vi "testIgnores Label Marker In Middle of Argument.vi"(8 "error in (no error)":errorcluster, 11 "TestCase in":refnum<class "Options Parsing Tests.lvclass">) -> (0 "error out":errorcluster, 3 "TestCase out":refnum<class "Options Parsing Tests.lvclass">)   [LabVIEW 2011, in "Options Parsing Tests.lvclass"]
uses:
  Options Parsing Tests.lvclass
  Argument Parser/Option Class/Option Configuration.ctl
  Argument Parser/Option Class/Argument Type.ctl
  <vilib>/addons/_JKI Toolkits/VI Tester/TestCase.llb/TestCase.lvclass
  Argument Parser/Option Set Class/Option Set.lvclass
  Argument Parser/Option Class/Option.lvclass
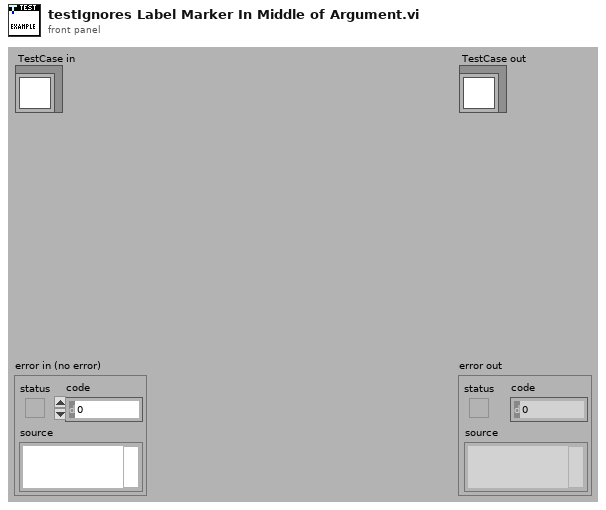
[diagram p1: front panel]
types:
  T1 = typedef "Option Parser.lvlib/Option.lvclass/Option Configuration.ctl" = cluster{"Option Type":T2, "Option Labels":string[], "Key":string, "Description":string, "Required":bool, "Default Value":string}
  T2 = typedef "Option Parser.lvlib/Option.lvclass/Argument Type.ctl" = enum16{"flag", "value"}
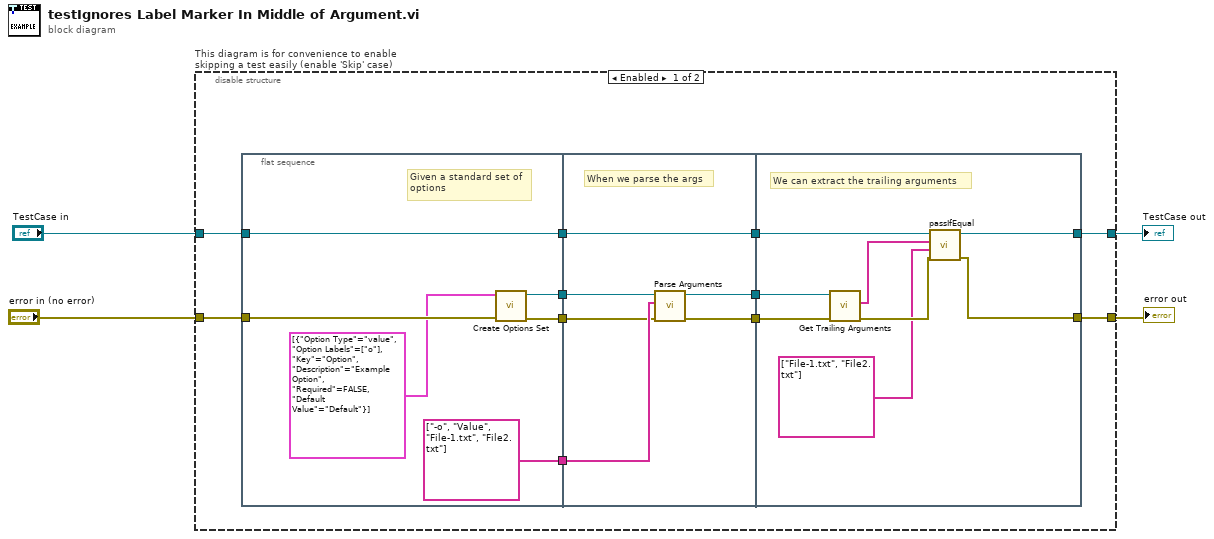
[diagram p0: block diagram]
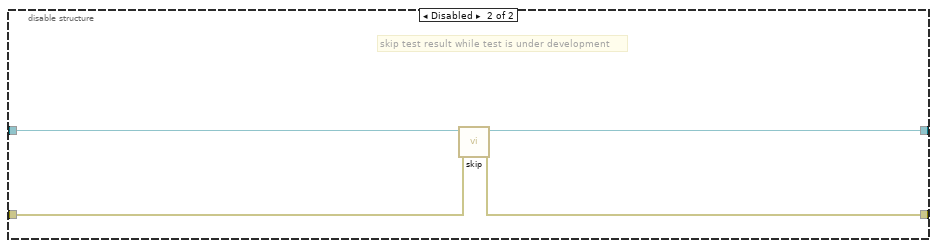
[diagram p2: hidden frame]
diagram:
  n1 = disable-structure "This diagram is for convenience to enable skipping a test easily (enable 'Skip' case)" shown="Enabled" {
    disable-tunnel: "TestCase in" -> [w7 w39]
    disable-tunnel: [w6 w37] -> w1
    disable-tunnel: [w5 w38] -> w3
    disable-tunnel: "error in (no error)" -> [w14 w36]
    frame Enabled {
      n2 = flat-sequence {
        tunnel: [string[] ["-o", "Value", "File-1.txt", "File2.txt"]] -> w15
        tunnel: w14 -> [w20]
        tunnel: [w19] -> w13
        tunnel: [w18] -> w12
        tunnel: [w17] -> w8
        tunnel: w7 -> [w17]
        tunnel: w15 -> [w27]
        tunnel: w13 -> [w26]
        tunnel: w12 -> [w25]
        tunnel: [w24] -> w11
        tunnel: [w23] -> w10
        tunnel: [w22] -> w9
        tunnel: w8 -> [w22]
        tunnel: w11 -> [w35]
        tunnel: w10 -> [w34]
        tunnel: w9 -> [w33]
        tunnel: [w29] -> w6
        tunnel: [w31] -> w5
        frame #0 {
          # "Given a standard set of\noptions"
          n3 = call "Create Options Set.vi"("error in (no error)"=w20, "Options"=T1[] [{"Option Type"=enum."value", "Option Labels"=["o"], "Key"="Option", "Description"="Example Option", "Required"=FALSE, "Default Value"="Default"}]) -> ("error out"=w19:errorcluster, "Option Set out"=w18:refnum<class "Option Set.lvclass">)  [unwired: 8 in]
        }
        frame #1 {
          # "When we parse the args"
          n4 = call "Parse Arguments.vi"("error in (no error)"=w26, "Arguments"=w27, "Option Set in"=w25) -> ("error out"=w23:errorcluster, "Option Set out"=w24:refnum<class "Option Set.lvclass">)  [unwired: 5 in, 2 out]
        }
        frame #2 {
          # "We can extract the trailing arguments"
          n5 = call "Get Trailing Arguments.vi"("error in (no error)"=w34, "Option Set in"=w35) -> ("error out"=w32:errorcluster, "Arguments"=w30:string[])  [unwired: 7 in, 1 out]
          n6 = call-dynamic "passIfEqual.vi"("error in (no error)"=w32, "y"=string[] ["File-1.txt", "File2.txt"], "x"=w30, "TestCase in"=w33) -> ("error out"=w31:errorcluster, "TestCase out"=w29:refnum<class "Options Parsing Tests.lvclass">)  [unwired: 6 in]
        }
      }
    }
    frame Disabled {
      # "skip test result while test is under development"
      n7 = call <vilib>:"skip.vi"("error in (no error)"=w36, "TestCase in"=w39) -> ("error out"=w38:errorcluster, "TestCase out"=w37:refnum<class "Options Parsing Tests.lvclass">)  [unwired: 8 in]
    }
  }
  "error out" <- w3
  "TestCase out" <- w1
